vi "VItoJPG.vi"(1 "name":string, 2 "Dest":path) -> (0 "appended path":path)   [LabVIEW 2012]
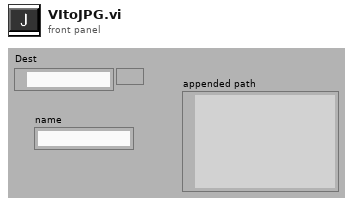
[diagram p1: front panel]
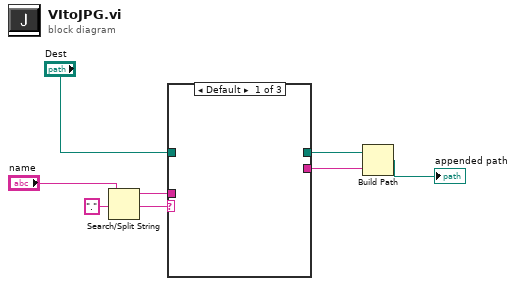
[diagram p0: block diagram]
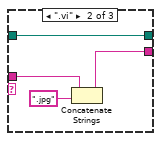
[diagram p2: hidden frame]
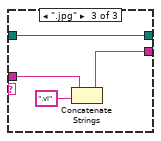
[diagram p3: hidden frame]
diagram:
  n1 = Search/Split String(string="name", search string/char (-)=".") -> (substring before match=w5:string, match + rest of string=w3:string)  [unwired: 1 in, 1 out]
  n2 = case shown="Default" w3 {
    tunnel: [_ w9 w13] -> w8
    tunnel: [_ w12 w16] -> w6
    tunnel: w5 -> [_ w10 w14]
    tunnel: "Dest" -> [_ w9 w13]
    frame Default {
    }
    frame ".vi" {
      n3 = Concatenate Strings(w10, ".jpg" ("search string/char (-)")) -> (w12:string)
    }
    frame ".jpg" {
      n4 = Concatenate Strings(w14, ".vi" ("search string/char (-)")) -> (w16:string)
    }
  }
  n5 = Build Path(base path=w8, name or relative path=w6) -> (appended path=→"appended path":path)
